vi "Waveform, Calculate Mean.vi"(0 "error in":errorcluster, 3 "waveform":waveform(dbl)={"t0"=timestamp(3473168073.631 s since 1904-01-01), "dt"=1e-08, "Y"=[], "attributes"=variant("Average Size"=variant(dbl 15.0), "NSamp"=variant(dbl 400000.0), "Resistance (ohms)"=variant(dbl 500.0), "Samp Freq (MHz)"=variant(dbl 100.0), "dt (us)"=variant(dbl 0.01))}, 4 "index":dbl[](array[numeric]) format="%0.2f") -> (7 "error out":errorcluster, 9 "mean (us)":dbl=nan format="%.3f", 10 "waveform dup":waveform(dbl)={"t0"=timestamp(-9593190233.15 s since 1904-01-01), "dt"=nan, "Y"=[], "attributes"=variant("Average Size"=variant(dbl 15.0), "NSamp"=variant(dbl 113636.0), "Resistance (ohms)"=variant(dbl 10000.0), "Samp Freq (MHz)"=variant(dbl 0.5), "dt (us)"=variant(dbl 2.0))})   [LabVIEW 2010]
doc: "Interphase Delay is measured between the Stimulus and Recovery pulses at points equal to 50% of the pulse amplitude. Results are stored as Waveform attributes and to an array of clusters."
uses:
  <vilib>/Analysis/NI_AALBase.lvlib
panel:
  out "mean index":dbl=nan format="%.3f"
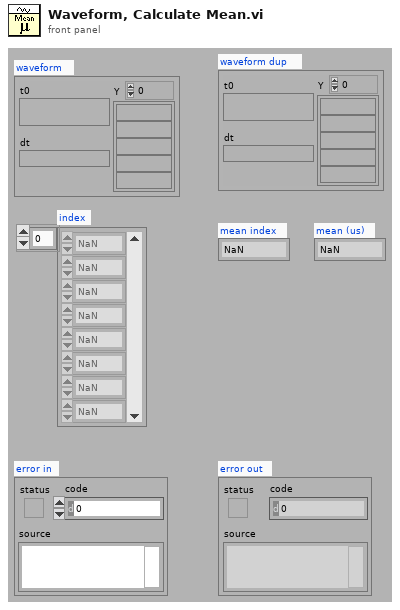
[diagram p1: front panel]
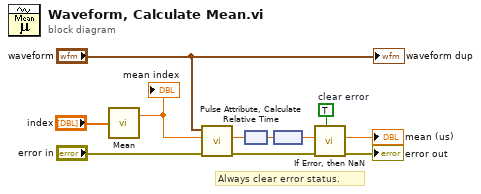
[diagram p0: block diagram]
diagram:
  w6 = TRUE  # clear error
  # "Always clear error status."
  n1 = call <vilib>:"Mean.vi"("X"="index") -> ("mean"=w1:dbl)  [unwired: 1 out]
  "mean index" <- w1
  n2 = call "Pulse Attribute, Calculate Relative Time.vi"("error in"="error in", "index"=w1, "waveform"="waveform") -> ("error out"=w3:errorcluster, "relative time (s)"=w2:dbl)  [unwired: 4 in, 1 out]
  n3 = node(w2) -> (w5:dbl[unit])
  n4 = node(w5) -> (w4:dbl)
  n5 = call "If Error, then NaN.vi"("clear error (F)"=w6, "error in (T)"=w3, "value2"=w4) -> ("error out"=→"error out":errorcluster, "value out2"=→"mean (us)":dbl)  [unwired: 3 in, 2 out]
  "waveform dup" <- "waveform"
